vi "TUNA Find red target.vi"(0 "Image In":T1, 1 "error in (no error)":errorcluster) -> (2 "Image Dst Out":T1, 3 "Nb Circles (Circle Detection 1)":i32, 4 "Camera Data":T2(array[cluster]), 5 "error out":errorcluster)   [LabVIEW 2014]
doc: "This VI takes in an image and finds a round, red target. It produces the target location and size."
uses:
  <vilib>/vision/Image Controls.llb/IMAQ Image.ctl
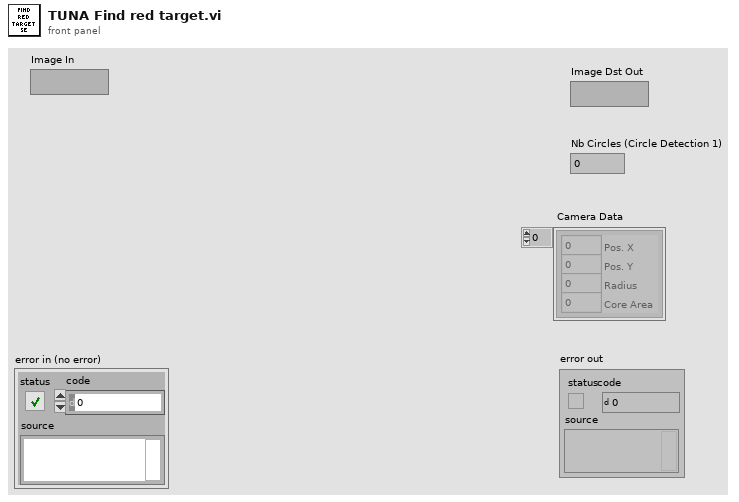
[diagram p1: front panel]
types:
  T1 = typedef "IMAQ Image.ctl" = refnum<image>
  T2 = cluster{"Pos. X":i32, "Pos. Y":i32, "Radius":i32, "Core Area":i32}[]
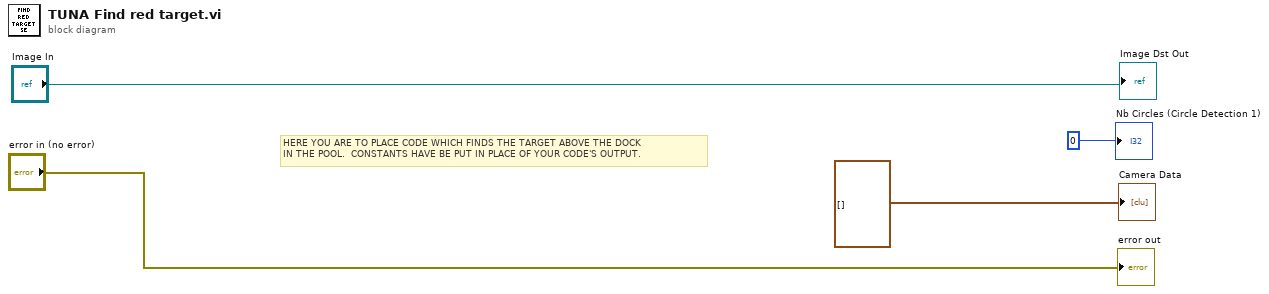
[diagram p0: block diagram]
diagram:
  # "HERE YOU ARE TO PLACE CODE WHICH FINDS THE TARGET ABOVE THE DOCK\nIN THE POOL.  CONSTANTS HAVE BE PUT IN PLACE OF YOUR CODE'S OUTPUT."
  "Nb Circles (Circle Detection 1)" <- 0
  "Camera Data" <- T2 [] ("Circles Data")
  "error out" <- "error in (no error)"
  "Image Dst Out" <- "Image In"
